vi "Video Processor main.vi"() -> ()   [LabVIEW 2018]
uses:
  Video Processor main Core Status Indicator STYP.ctl
  Video Processor main Status STYP.ctl
  Video Processor main Core Status STYP.ctl
  Video Processor main File Status STYP.ctl
  <userlib>/Jet Engineering/JET_QSM/Code/Private/JET_QSM_InvalidOption STYP.ctl
  <userlib>/Jet Engineering/JET_QSM/Code/Private/JET_QSM - Add State [String API].vi
  80037c5a-716f-4bc2-9a3a-c8c93484ebcc.vi
  35257932-e252-4286-8d59-1e758d2cb38c.vi
  <vilib>/Utility/error.llb/Trim Whitespace.vi
  <vilib>/Utility/error.llb/Error Cluster From Error Code.vi
panel:
  out "Core Statuses":T1[](array[typedef]) {"Progress" scale=0.0..100.0}
  out "Converting?":bool
  out "Progress":dbl(slide) scale=0.0..100.0
  in  "Convert":bool
  in  "Folder":path
  out "Recent states before Error (with tick counts) 2":string="0.167 sec ago: VI Initialize\n0.167 sec ago: Window Open\n0.110 sec ago: Control Update\n0.110 sec ago: Indicator Update\n0.000 sec ago: Error Handler\r\n"
  out "error out":errorcluster
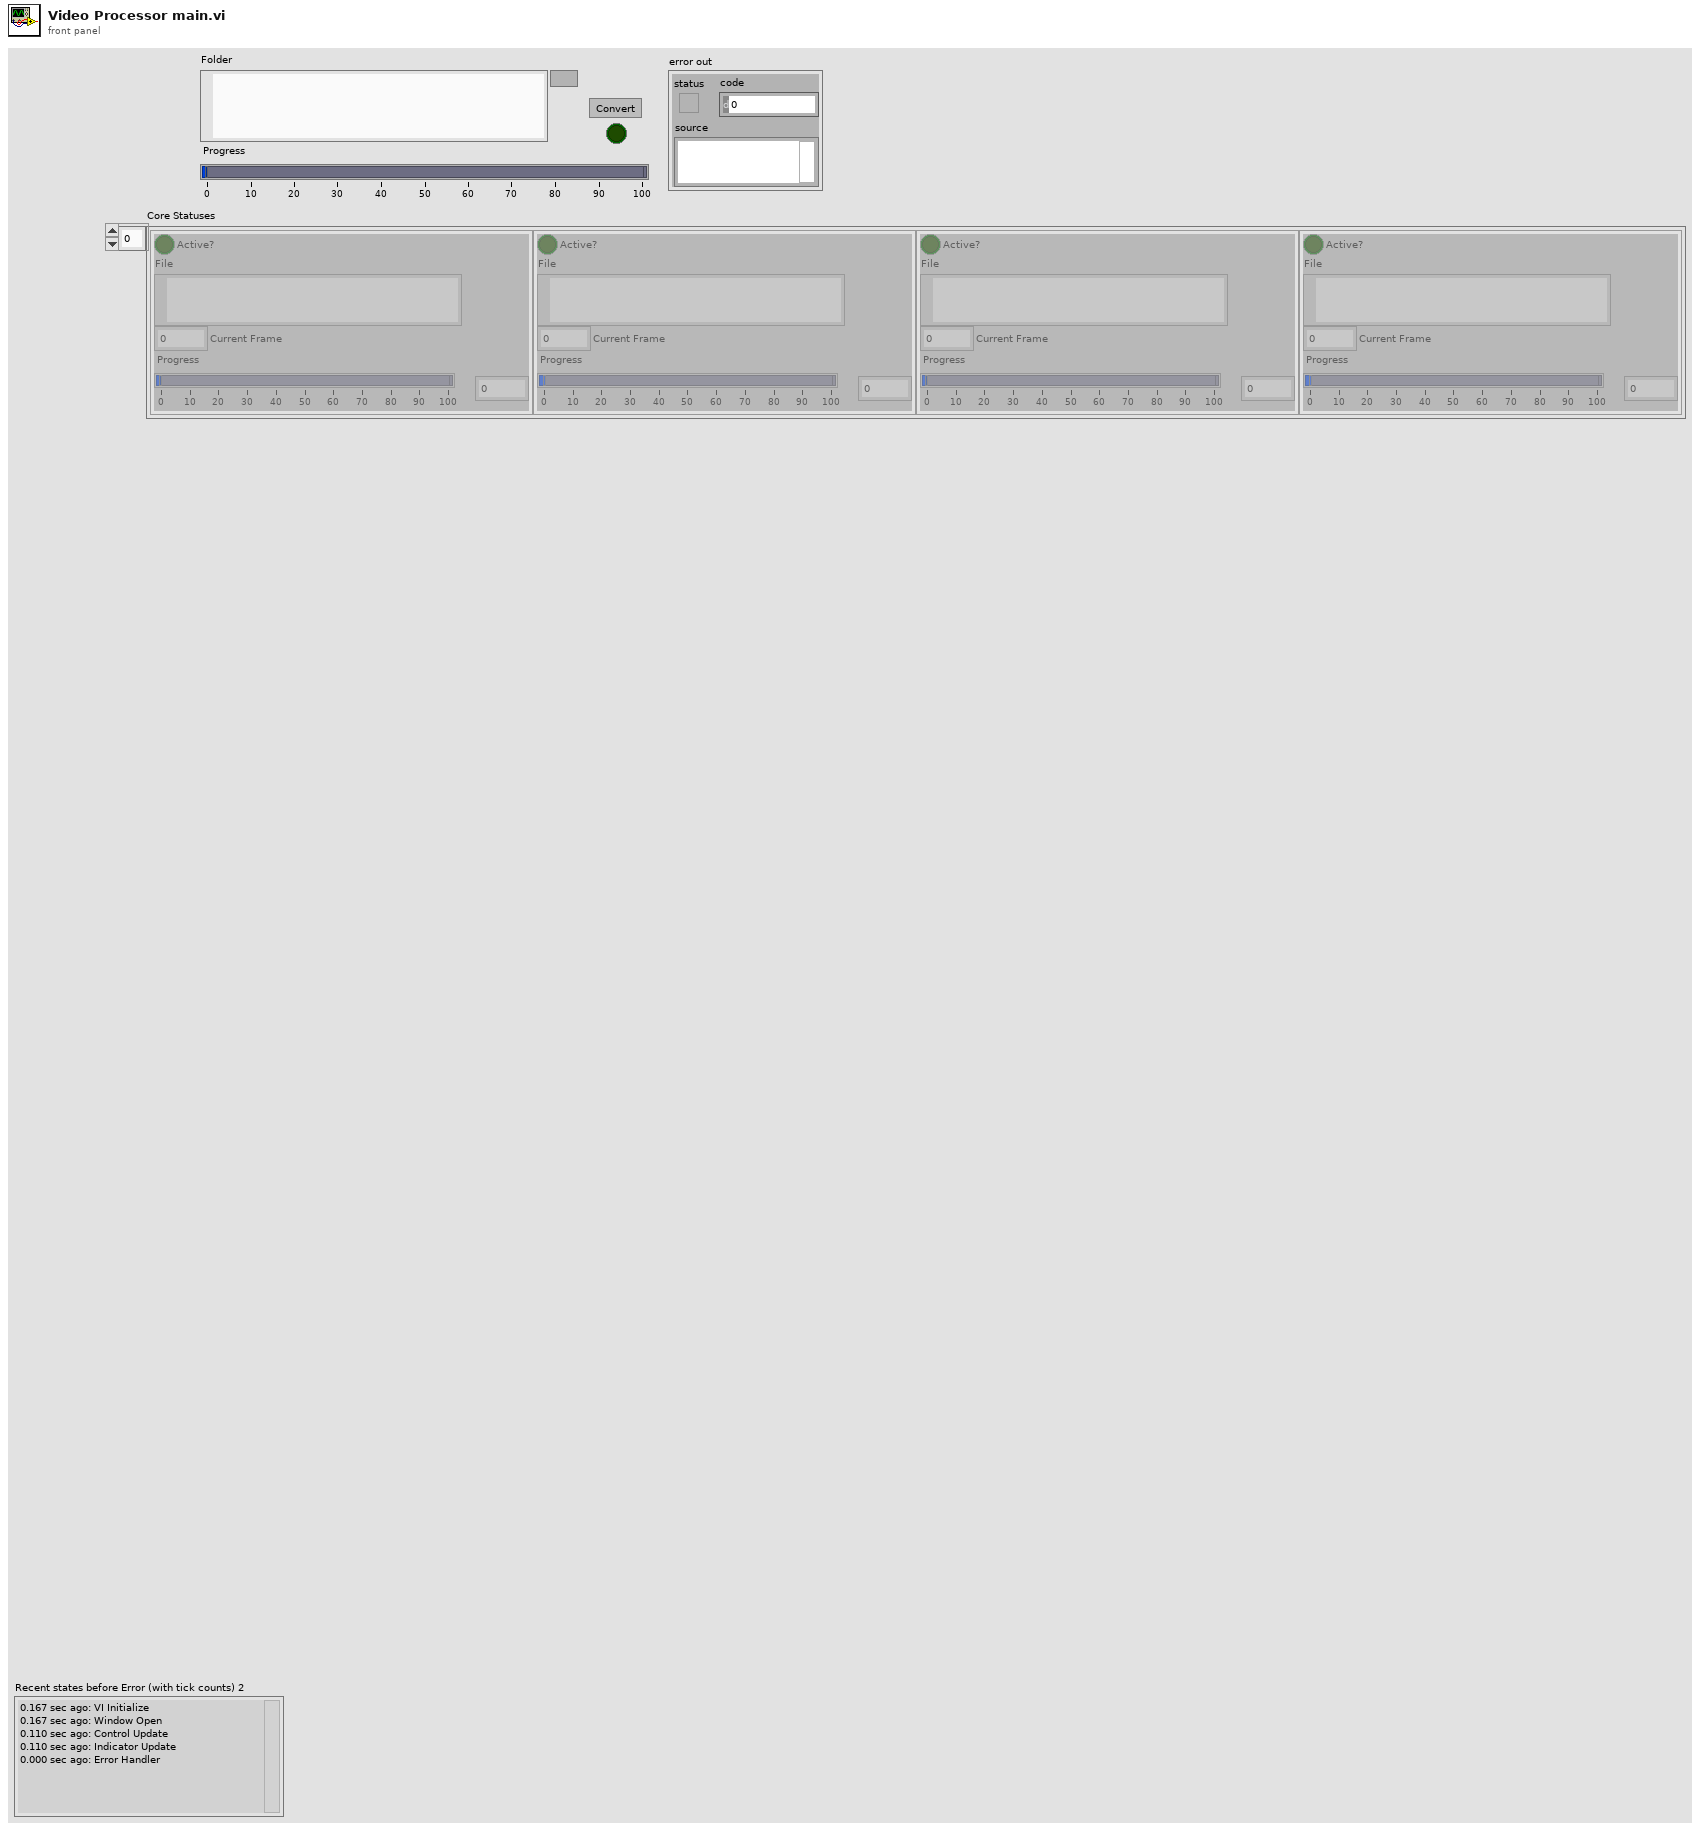
[diagram p1: front panel]
types:
  T1 = typedef "Video Processor main Core Status Indicator STYP.ctl" = cluster{"Active?":bool, "File":path, "Current Frame":i32, "Progress":dbl}
  T2 = typedef "Video Processor main Status STYP.ctl" = cluster{"VI":cluster{"error":errorcluster, "isExiting?":bool}, "UserLoggedIn?":bool, "Converting?":bool, "Input Folder":path, "Files":path[], "Files Complete":i32, "Total File Count":i32, "Core Status":T3[], "Events":cluster{"Refnum":refnum<event-registration>, "Core Release Event":refnum<user-event>, "File Status Event":refnum<user-event>}}
  T3 = typedef "Video Processor main Core Status STYP.ctl" = cluster{"Active?":bool, "File":path, "Current Frame":u32, "Total Frames":u32}
  T4 = typedef "JET_QSM_InvalidOption STYP.ctl" = enum16{"Ignore", "Dialog", "Error"}
  T5 = typedef "JET_QSM_Refnum STYP.ctl" = cluster{"state":cluster{"queue":refnum<queue>, "idle":string, "error":string, "STOP":string}, "debug":cluster{"enabled?":bool, "queue":refnum<queue>}, "Invalid.option":T4, "QSM.Name":string}
  T6 = enum32{"invalid app kind", "Development System", "Run Time System", "Student Edition", "Embedded LabVIEW", "Evaluation", "Custom"}
  T7 = typedef "Video Processor main File Status STYP.ctl" = cluster{"Index":i32, "Current Frame":u32, "Total Frames":u32}
  T8 = typedef "JET_QSM_Element STYP.ctl" = cluster{"state":string, "data":variant, "comment":string}
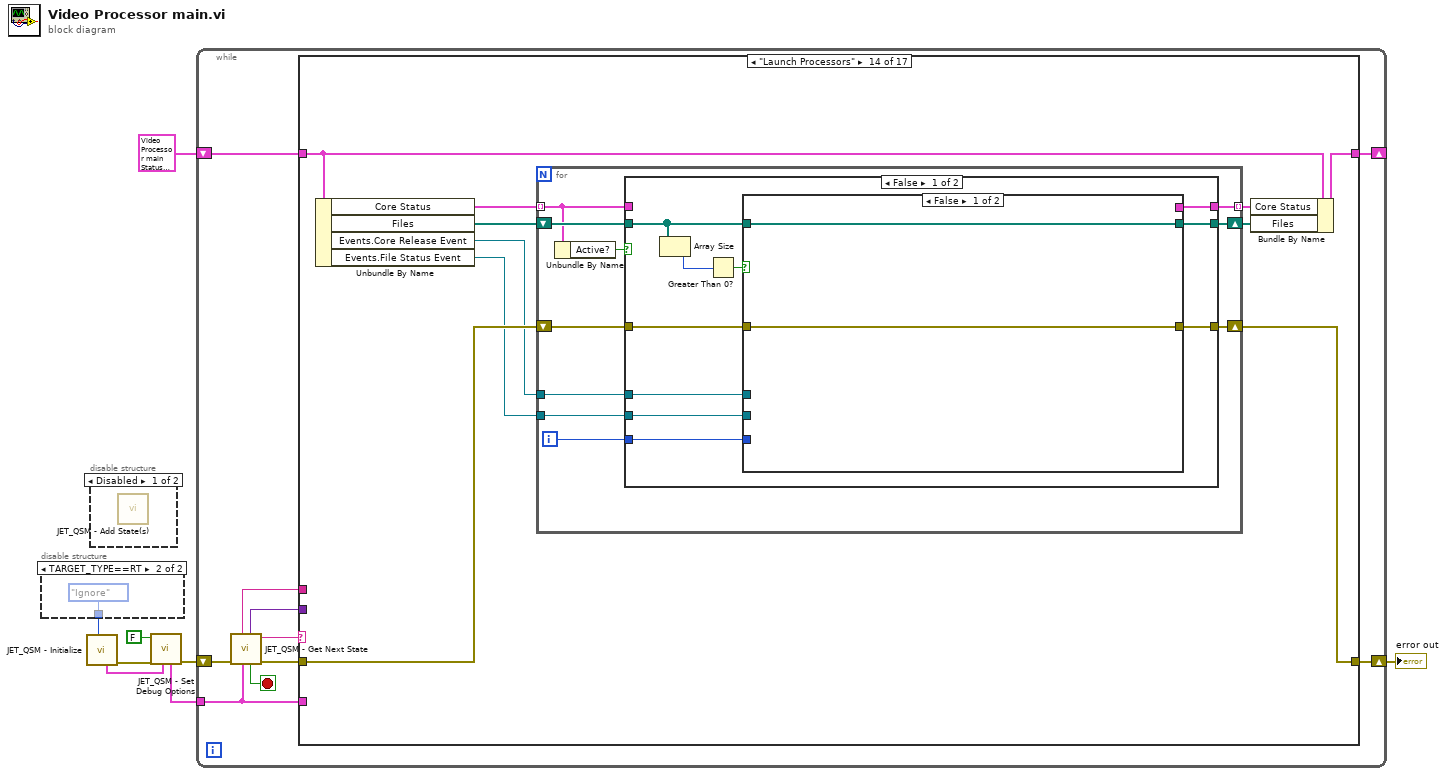
[diagram p0: block diagram]
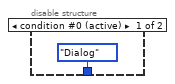
[diagram p2: hidden frame]
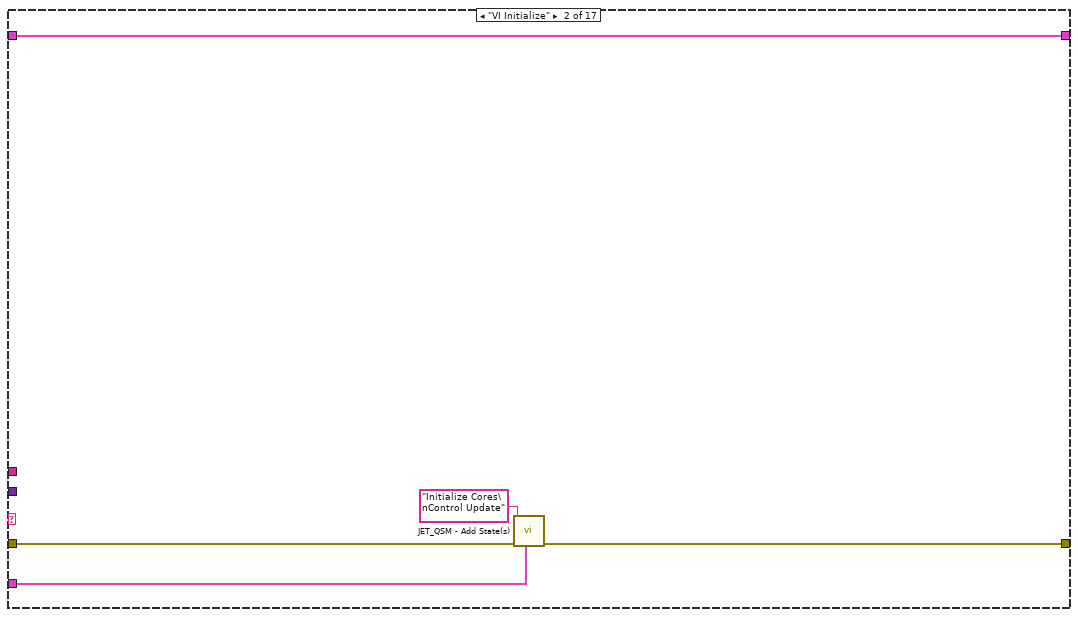
[diagram p5: hidden frame]
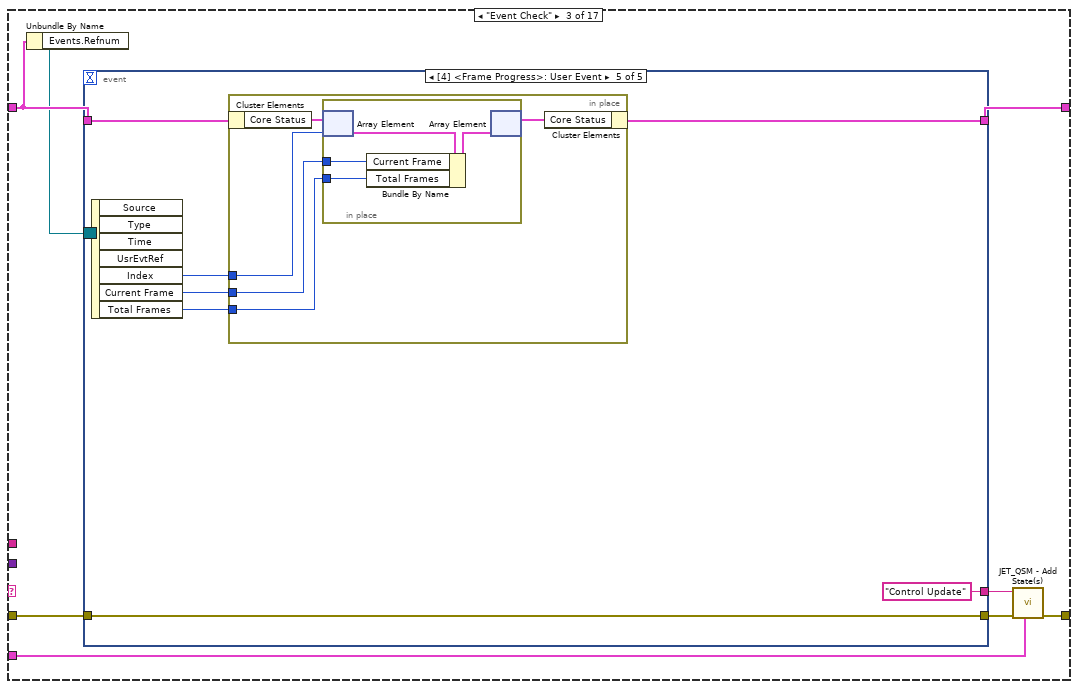
[diagram p6: hidden frame]
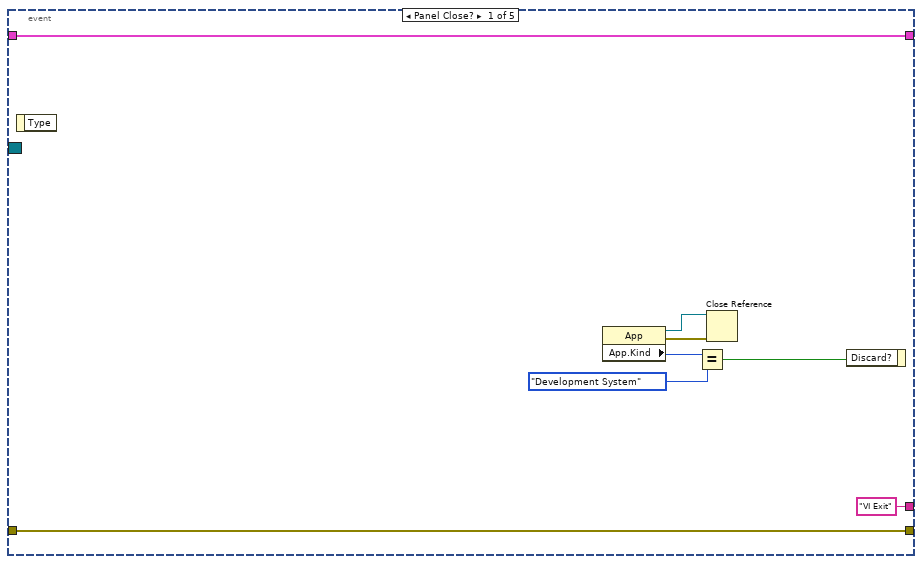
[diagram p7: hidden frame]
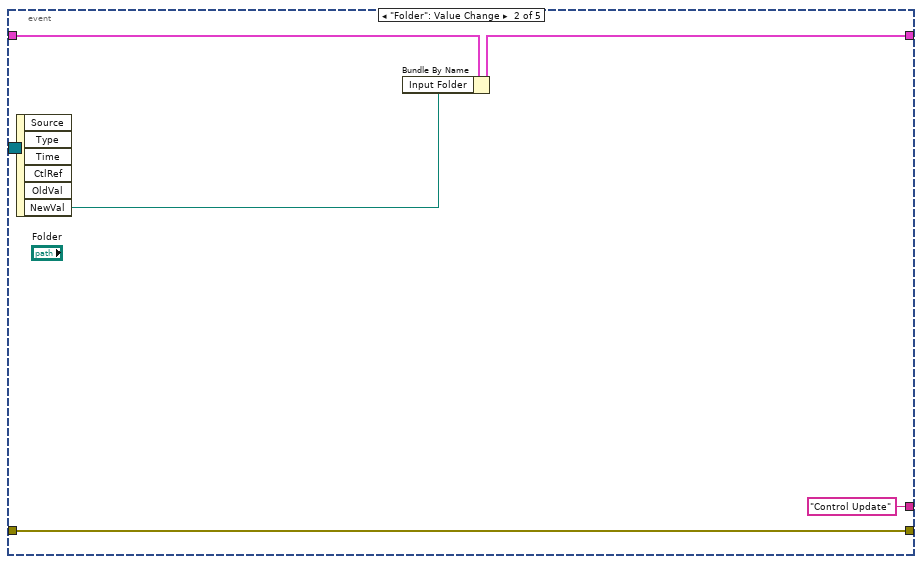
[diagram p8: hidden frame]
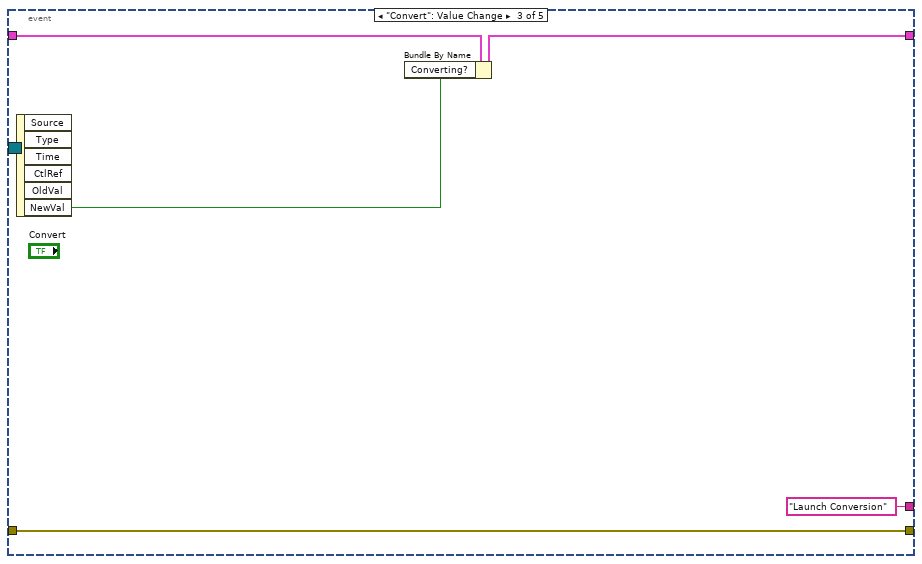
[diagram p9: hidden frame]
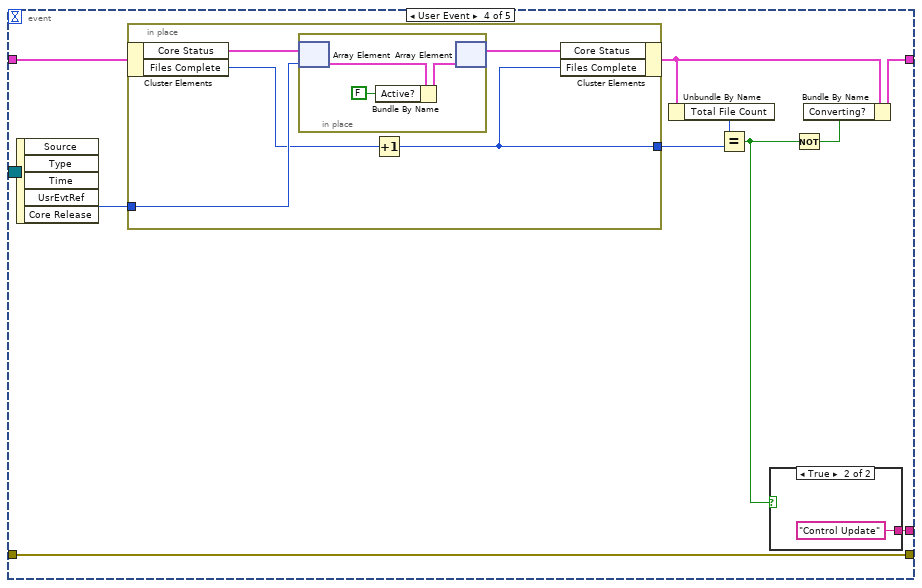
[diagram p10: hidden frame]
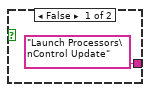
[diagram p11: hidden frame]
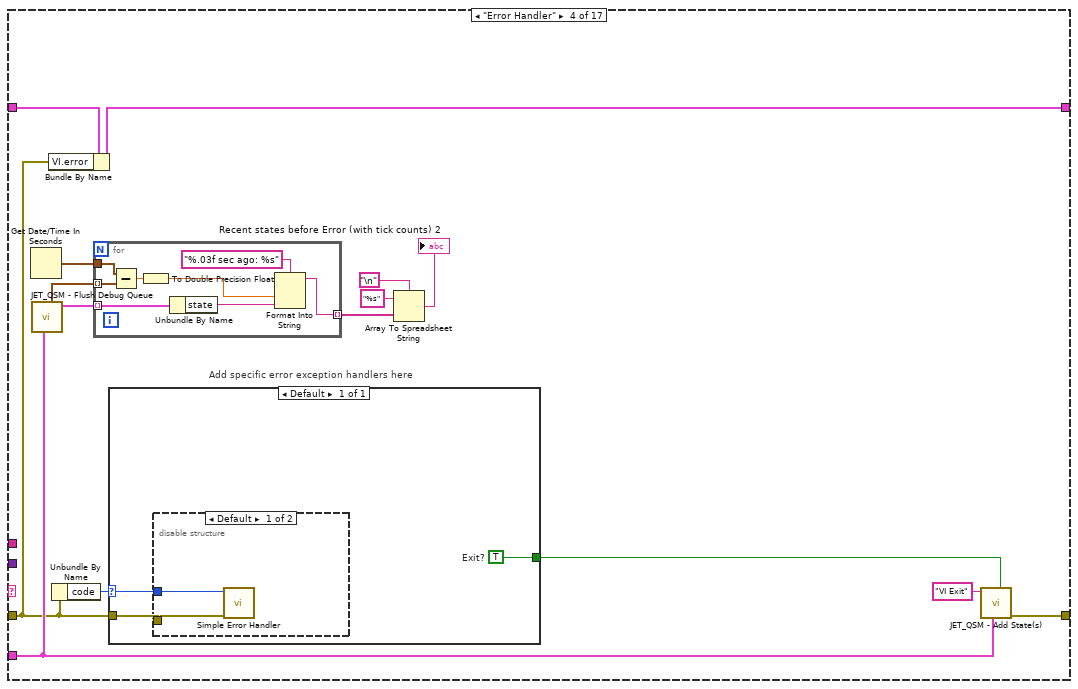
[diagram p12: hidden frame]
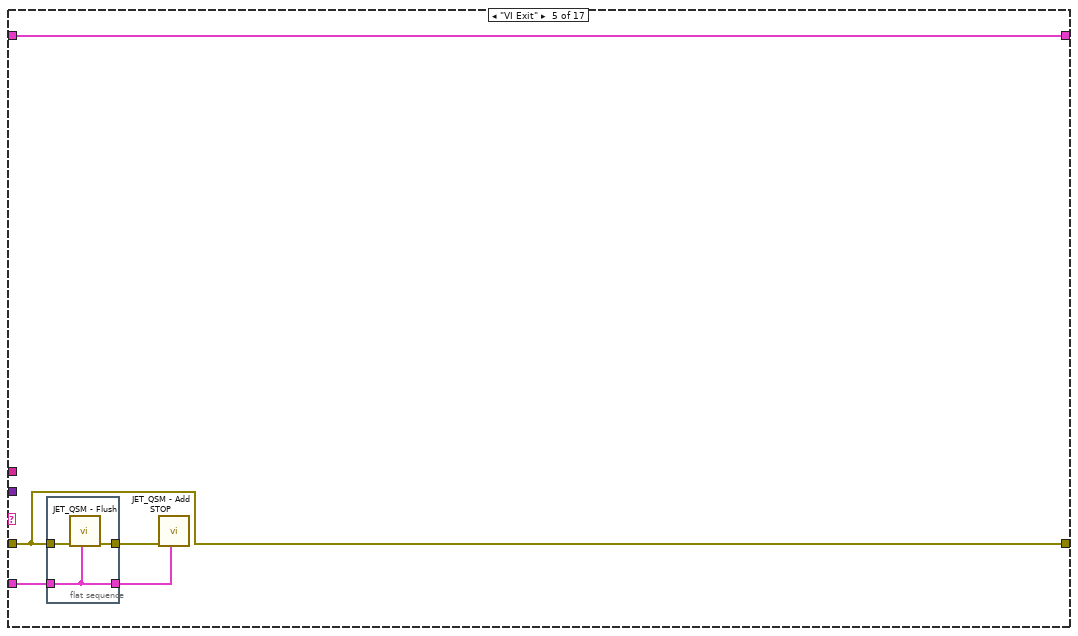
[diagram p14: hidden frame]
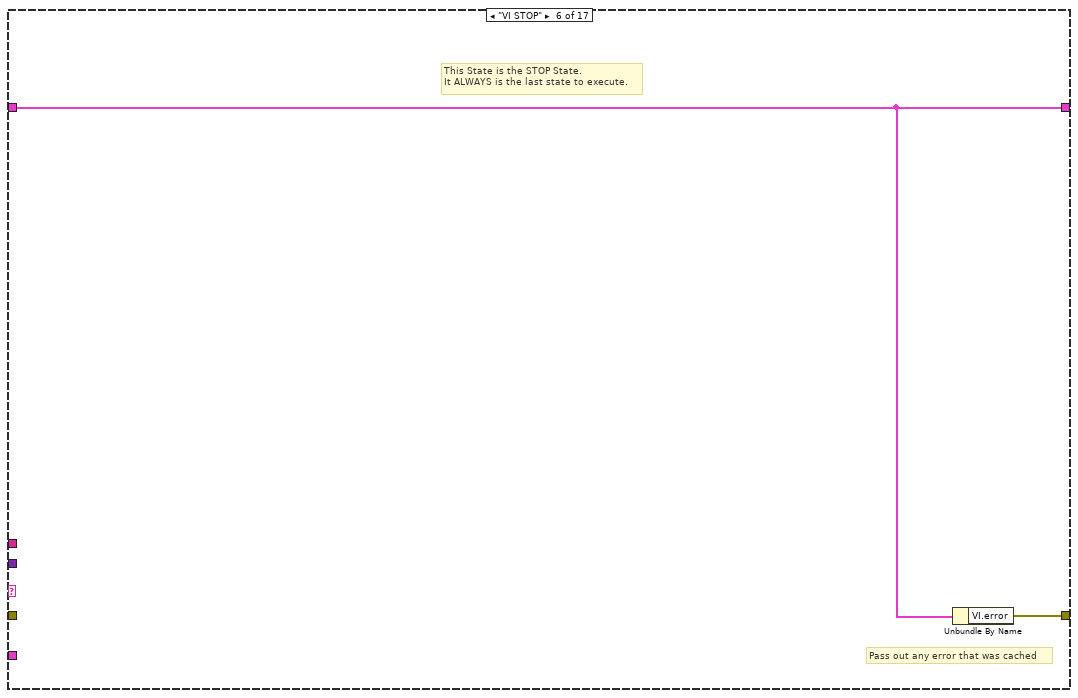
[diagram p15: hidden frame]
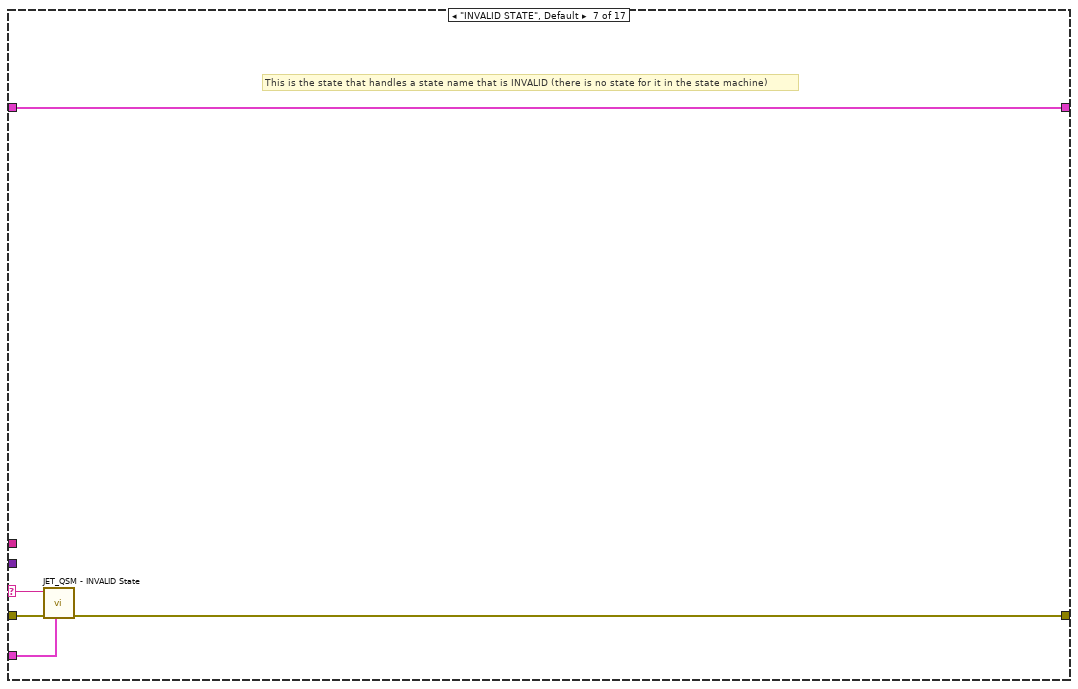
[diagram p16: hidden frame]
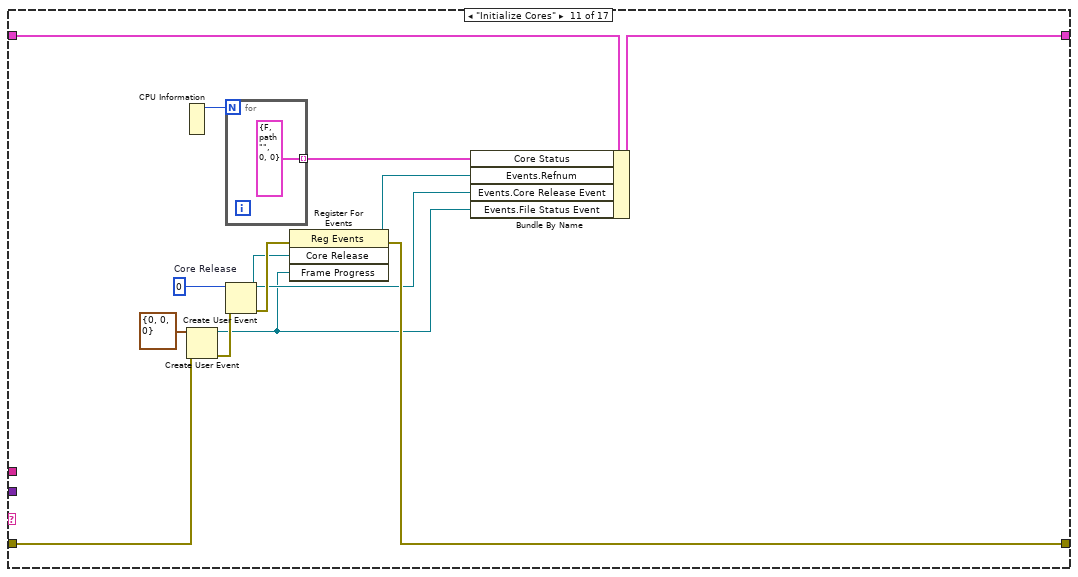
[diagram p20: hidden frame]
diagram:
  n1 = disable-structure shown="TARGET_TYPE==RT" {
    disable-tunnel: [JET_QSM_InvalidOption_STYP."Dialog" ("invalid state action (Dialog)") JET_QSM_InvalidOption_STYP."Ignore" ("invalid state action (Dialog)")] -> w8
    frame condition #0 (active) {
    }
    frame condition #1 {
    }
  }
  n2 = call <userlib>:"JET_QSM - Initialize.vi"("invalid state action (Dialog)"=w8) -> ("error out"=w1:errorcluster, "Jet_QSM refnum"=w4:T5)  [unwired: 9 in]
  n3 = disable-structure shown="Disabled" {
    frame Disabled {
      n4 = call-poly <userlib>:"JET_QSM - Add State(s).vi"() -> ()  [unwired: 11 in, 1 out]
    }
    frame Enabled {
    }
  }
  n5 = call <userlib>:"JET_QSM - Set Debug Options.vi"("Jet_QSM refnum"=w4, "error in (no error)"=w1, "debug.enabled? (F)"=FALSE) -> ("error out"=w2:errorcluster, "Jet_QSM ref"=w3:T5)  [unwired: 7 in]
  n6 = while {
    tunnel: w3 -> [w16]
    shift-right: [w14] -> _
    shift-left: T2 {"VI"={"error"={"status"=FALSE, "code"=0, "source"=""}, "isExiting?"=FALSE}, "UserLoggedIn?"=FALSE, "Converting?"=FALSE, "Input Folder"=path "", "Files"=[], "Files Complete"=0, "Total File Count"=0, "Core Status"=[], "Events"={"Refnum"=refnum, "Core Release Event"=refnum, "File Status Event"=refnum}} ("Status") -> [w15]
    shift-right: [w13] -> w7
    shift-left: w2 -> [w20]
    stop <- w17 stop-if-true
    n7 = call <userlib>:"JET_QSM - Get Next State.vi"("Jet_QSM refnum"=w16, "error in (no error)"=w20) -> ("error out"=w19:errorcluster, "state"=w18:string, "Stop Loop?"=w17:bool, "state data"=w12:variant, "state comment"=w11:string)  [unwired: 5 in]
    n8 = case shown="\"Launch Processors\"" w18 {
      selector: w18 -> [_ _ _ _ _ _ w130 _ _ _ _ _ _ _ _ _ _]
      tunnel: w19 -> [w21 w26 w35 w91 w122 _ w131 w133 w135 w137 w142 w156 w166 w177 w221 w229 w238]
      tunnel: w16 -> [_ w24 w34 w96 w120 _ w129 _ _ _ _ w154 _ _ _ w230 _]
      tunnel: w15 -> [w22 w27 w29 w92 w118 w126 w132 w134 w136 w138 w150 w157 w162 w173 w222 w227 w237]
      tunnel: [w22 w27 w30 w90 w118 w126 w132 w134 w136 w138 w144 w157 w161 w170 w222 w227 w237] -> w14
      tunnel: [w21 w25 w32 w97 w122 w127 w128 w133 w135 w137 w146 w155 w165 w176 w221 w228 w238] -> w13
      tunnel: w12 -> [_ _ _ _ _ _ _ _ _ _ _ _ _ _ _ _ _]
      tunnel: w11 -> [_ _ _ _ _ _ _ _ _ _ _ _ _ _ _ _ _]
      frame "------ Standard States ------" {
        # "Standard States are required states for a JET_QSM State Machine\n\nTheir names may be changed; use the Initialize function to specify the new names"
        # "This is a section header; the state is never expected to execute"
      }
      frame "VI Initialize" {
        n9 = call-poly <userlib>:"JET_QSM - Add State(s).vi"("Jet_QSM refnum"=w24, "error in (no error)"=w26, "state(s)"="Initialize Cores\nControl Update") -> ("error out"=w25:errorcluster)  [unwired: 8 in]
      }
      frame "Event Check" {
        n10 = Unbundle By Name(w29) -> ("Events.Refnum"=w28:refnum<event-registration>)
        n11 = event shown="[4] <Frame Progress>: User Event" {
          selector: w28 -> [_ _ _ _ _]
          dyn-events: _ -> [_ _ _ _ _]
          timeout: _ -> [_ _ _ _ _]
          tunnel: w35 -> [w37 w48 w53 w61 w75]
          tunnel: ["VI Exit" ("state(s)") "Control Update" ("state(s)") "Launch Conversion" ("state(s)") w60 "Control Update" ("state(s)")] -> w33
          tunnel: [w37 w48 w53 w61 w75] -> w31
          tunnel: w29 -> [w36 w46 w51 w63 w80]
          tunnel: [w36 w45 w49 w56 w79] -> w30
          event Panel Close? {
            n12 = event-data() -> ()  [unwired: 1 in, 1 out]
            n13 = property class="App"() -> (reference out=w39:refnum<vi>, error out=w40:errorcluster, "App.Kind"=w43:T6)  [unwired: 2 in]
            n14 = Equal?(x=w43, y=T6."Development System") -> (x = y?=w41:bool)
            n15 = Close Reference(reference=w39, error in (no error)=w40) -> ()  [unwired: 1 out]
            n16 = event-data("Discard?"=w41) -> ()  [unwired: 1 in, 1 out]
          }
          event "Folder": Value Change {
            n17 = event-data() -> ("NewVal"=w44:path)  [unwired: 1 in, 5 out]
            n18 = Bundle By Name(cluster=w46, "Input Folder"=w44) -> (w45:T2)
          }
          event "Convert": Value Change {
            n19 = event-data() -> ("NewVal"=w50:bool)  [unwired: 1 in, 5 out]
            n20 = Bundle By Name(cluster=w51, "Converting?"=w50) -> (w49:T2)
          }
          event User Event {
            n21 = event-data() -> ("Core Release"=w62:i32)  [unwired: 1 in, 4 out]
            n22 = in-place {
              in-place-border: w62 -> [w69]
              in-place-border: [w66] -> w58
              n23 = in-place-cluster #1(w63) -> ("Core Status"=w70:T3[], "Files Complete"=w67:i32)
              n24 = in-place {
                n25 = in-place-array #2(w70, w69) -> (w73:T3)
                n26 = Bundle By Name(cluster=w73, "Active?"=FALSE) -> (w71:T3)
                n27 = in-place-array #2(w71) -> (w68:T3[])  [unwired: 1 out]
              }
              n28 = Increment(x=w67) -> (x+1=w66:i32)
              n29 = in-place-cluster #1("Core Status"=w68, "Files Complete"=w66) -> (w57:T2)
            }
            n30 = Unbundle By Name(w57) -> ("Total File Count"=w59:i32)
            n31 = Equal?(x=w59, y=w58) -> (x = y?=w54:bool)
            n32 = case shown="True" w54 {
              tunnel: ["Launch Processors\nControl Update" ("state(s)") "Control Update" ("state(s)")] -> w60
              frame False {
              }
              frame True {
              }
            }
            n33 = Not(x=w54) -> (.not. x?=w55:bool)
            n34 = Bundle By Name(cluster=w57, "Converting?"=w55) -> (w56:T2)
          }
          event User Event {
            n35 = event-data() -> ("Index"=w78:i32, "Current Frame"=w77:u32, "Total Frames"=w76:u32)  [unwired: 1 in, 4 out]
            n36 = in-place {
              in-place-border: w78 -> [w83]
              in-place-border: w77 -> [w82]
              in-place-border: w76 -> [w81]
              n37 = in-place-cluster #3(w80) -> ("Core Status"=w85:T3[])
              n38 = in-place {
                in-place-border: w82 -> [w88]
                in-place-border: w81 -> [w87]
                n39 = in-place-array #4(w85, w83) -> (w89:T3)
                n40 = Bundle By Name(cluster=w89, "Current Frame"=w88, "Total Frames"=w87) -> (w86:T3)
                n41 = in-place-array #4(w86) -> (w84:T3[])  [unwired: 1 out]
              }
              n42 = in-place-cluster #3("Core Status"=w84) -> (w79:T2)
            }
          }
        }
        n43 = call-poly <userlib>:"JET_QSM - Add State(s).vi"("Jet_QSM refnum"=w34, "error in (no error)"=w31, "state(s)"=w33) -> ("error out"=w32:errorcluster)  [unwired: 8 in]
      }
      frame "Error Handler" {
        # "Add specific error exception handlers here"
        n44 = Get Date/Time In Seconds() -> (seconds since 1Jan1904=w100:timestamp)
        n45 = call <userlib>:"JET_QSM - Flush Debug Queue.vi"("Jet_QSM refnum"=w96) -> ("QSM Elements"=w98:T8[], "Timestamps"=w99:timestamp[])  [unwired: 8 in, 1 out]
        n46 = Bundle By Name(cluster=w92, "VI.error"=w91) -> (w90:T2)
        n47 = Unbundle By Name(w91) -> ("code"=w93:i32)
        n48 = for {
          tunnel: w98 -> [w112] mode=indexing
          tunnel: [w110] -> w102 mode=indexing
          tunnel: w100 -> [w107]
          tunnel: w99 -> [w108] mode=indexing
          n49 = Subtract(x=w107, y=w108) -> (x-y=w106:dbl)
          n50 = To Double Precision Float(number=w106) -> (double precision float=w105:dbl)
          n51 = Unbundle By Name(w112) -> ("state"=w111:string)
          n52 = Format Into String(format string="%.03f sec ago: %s", w105, w111) -> (resulting string=w110:string)  [unwired: 2 in, 1 out]
        }
        n53 = case shown="Default" w93 {
          selector: w93 -> [w114]
          tunnel: [w115] -> w94
          tunnel: w91 -> [w113]
          frame Default {
            w115 = TRUE  # Exit?
            n54 = disable-structure shown="Default" {
              disable-tunnel: w114 -> [w117 _]
              disable-tunnel: w113 -> [w116 _]
              frame condition #0 (active) {
                n55 = call <vilib>:"Simple Error Handler.vi"("error code (no error:0)"=w117, "error in (no error)"=w116) -> ()  [unwired: 3 in, 5 out]
              }
              frame condition #1 {
              }
            }
          }
        }
        n56 = Array To Spreadsheet String(delimiter (Tab)="\n", array=w102, 3:"%s" ("format string")) -> (spreadsheet string=→"Recent states before Error (with tick counts) 2":string)
        n57 = call-poly <userlib>:"JET_QSM - Add State(s).vi"("act? (T)"=w94, "Jet_QSM refnum"=w96, "state(s)"="VI Exit") -> ("error out"=w97:errorcluster)  [unwired: 8 in]
      }
      frame "VI Exit" {
        n58 = flat-sequence {
          tunnel: w122 -> [w125]
          tunnel: [w124] -> w121
          tunnel: w120 -> [w123]
          tunnel: [w123] -> w119
          frame #0 {
            n59 = call <userlib>:"JET_QSM - Flush.vi"("Jet_QSM ref"=w123, "error in (no error)"=w125) -> ("error out"=w124:errorcluster)  [unwired: 8 in, 1 out]
          }
        }
        n60 = call <userlib>:"JET_QSM - Add STOP.vi"("Jet_QSM refnum"=w119, "error in (no error)"=w121) -> ()  [unwired: 9 in, 1 out]
      }
      frame "VI STOP" {
        # "Pass out any error that was cached"
        # "This State is the STOP State.\nIt ALWAYS is the last state to execute."
        n61 = Unbundle By Name(w126) -> ("VI.error"=w127:errorcluster)
      }
      frame "INVALID STATE", Default {
        # "This is the state that handles a state name that is INVALID (there is no state for it in the state machine)"
        n62 = call <userlib>:"JET_QSM - INVALID State.vi"("Jet_QSM refnum"=w129, "error in (no error)"=w131, "state"=w130) -> ("error out"=w128:errorcluster)  [unwired: 8 in]
      }
      frame "------ Menu Commands ------" {
        # "This is a section header; the state is never expected to execute"
      }
      frame "------ Events  ------" {
        # "This is a section header; the state is never expected to execute"
      }
      frame "------ Actions  ------" {
        # "This is a section header; the state is never expected to execute"
      }
      frame "Initialize Cores" {
        w148 = 0  # Core Release
        n63 = CPU Information() -> (4:w151:i32)  [unwired: 3 out]
        n64 = Create User Event(user event datatype=T7 {"Index"=0, "Current Frame"=0, "Total Frames"=0} ("Frame Progress"), error in=w142) -> (user event=w139:refnum<user-event>, error out=w141:errorcluster)
        n65 = for {
          N: w151 -> [_]
          tunnel: [T3 {"Active?"=FALSE, "File"=path "", "Current Frame"=0, "Total Frames"=0} ("Core")] -> w149 mode=indexing
        }
        n66 = Create User Event(user event datatype=w148, error in=w141) -> (user event=w143:refnum<user-event>, error out=w147:errorcluster)
        n67 = register-events(error in=w147, w143, w139) -> (reference out=w145:refnum<event-registration>, error out=w146:errorcluster)  [unwired: 1 in]
        n68 = Bundle By Name(cluster=w150, "Core Status"=w149, "Events.Refnum"=w145, "Events.Core Release Event"=w143, "Events.File Status Event"=w139) -> (w144:T2)
      }
      frame "Launch Conversion" {
        n69 = call-poly <userlib>:"JET_QSM - Add State(s).vi"("Jet_QSM refnum"=w154, "error in (no error)"=w156, "state(s)"="Find Files\nLaunch Processors\nControl Update") -> ("error out"=w155:errorcluster)  [unwired: 8 in]
      }
      frame "Find Files" {
        n70 = Unbundle By Name(w162) -> ("Input Folder"=w164:path)
        n71 = List Folder(path=w164, error in=w166) -> (filenames=w163:string[], error out=w165:errorcluster)  [unwired: 2 in, 2 out]
        n72 = for {
          tunnel: w164 -> [w169]
          tunnel: w163 -> [w168] mode=indexing
          tunnel: [w167] -> w159 mode=indexing
          n73 = Build Path(base path=w169, name or relative path=w168) -> (appended path=w167:path)
        }
        n74 = Array Size(array=w159) -> (size(s)=w160:i32)
        n75 = Bundle By Name(cluster=w162, "Files"=w159, "Files Complete"=1, "Total File Count"=w160) -> (w161:T2)
      }
      frame "Launch Processors" {
        n76 = Unbundle By Name(w173) -> ("Core Status"=w179:T3[], "Files"=w178:path[], "Events.Core Release Event"=w175:refnum<user-event>, "Events.File Status Event"=w174:refnum<user-event>)
        n77 = for {
          tunnel: w179 -> [w187] mode=indexing
          shift-right: [w186] -> w171
          shift-left: w178 -> [w188]
          tunnel: [w185] -> w172 mode=indexing
          shift-right: [w183] -> w176
          shift-left: w177 -> [w184]
          tunnel: w175 -> [w182]
          tunnel: w174 -> [w181]
          i -> [w180]
          n78 = Unbundle By Name(w187) -> ("Active?"=w189:bool)
          n79 = case shown="False" w189 {
            tunnel: w188 -> [w192 w220]
            tunnel: w187 -> [_ w219]
            tunnel: [w199 w220] -> w186
            tunnel: [w193 w219] -> w185
            tunnel: w184 -> [w198 w218]
            tunnel: [w197 w218] -> w183
            tunnel: w182 -> [w195 _]
            tunnel: w181 -> [w196 _]
            tunnel: w180 -> [w194 _]
            frame False {
              n80 = Array Size(array=w192) -> (size(s)=w190:i32)
              n81 = Greater Than 0?(x=w190) -> (x > 0?=w191:bool)
              n82 = case shown="False" w191 {
                tunnel: w192 -> [w201 w217]
                tunnel: [w201 w216] -> w199
                tunnel: w198 -> [w200 w209]
                tunnel: [w200 w208] -> w197
                tunnel: w196 -> [_ w207]
                tunnel: w195 -> [_ w206]
                tunnel: w194 -> [_ w205]
                tunnel: [_ w202] -> w193
                frame False {
                }
                frame True {
                  n83 = Delete From Array(array=w217) -> (deleted portion=w203:path, array with subset deleted=w216:path[])  [unwired: 2 in]
                  n84 = vi-ref "Headless Modular Test W Events.vi"() -> (w212:refnum<vi>)
                  n85 = property class="VI Interface Type 0"(reference=w212, error in=w209) -> (error out=w215:errorcluster, "Path"=w214:path)  [unwired: 1 out]
                  n86 = Open VI Reference(type specifier VI Refnum (for type only)=w212, vi path=w214, options=128, error in (no error)=w215) -> (vi reference=w211:refnum<vi>, error out=w210:errorcluster)  [unwired: 2 in]
                  n87 = call-by-ref "Start Asynchronous Call"(reference=w211, error in=w210, "Core Index"=w205, "File Finished Event"=w206, "File Status Event"=w207, "Path"=w203) -> (error out=w208:errorcluster)  [unwired: 8 in, 1 out]
                  n88 = Bundle By Name(cluster=T3 {"Active?"=TRUE, "File"=path "", "Current Frame"=0, "Total Frames"=100} ("Core"), "File"=w203) -> (w202:T3)
                }
              }
            }
            frame True {
            }
          }
        }
        n89 = Bundle By Name(cluster=w173, "Core Status"=w172, "Files"=w171) -> (w170:T2)
      }
      frame "------ Window and Panel Control ------" {
        # "This is a section header; the state is never expected to execute"
      }
      frame "Control Update" {
        # "Update all control properties here from the status cluster\n(Consolidate/reduce property nodes)"
        n90 = Unbundle By Name(w227) -> ("Input Folder"=w225:path)
        n91 = call <vilib>:"Is Path and Not Empty.vi"("path"=w225) -> ("Is Path and Not Empty?"=w224:bool)  [unwired: 4 in]
        n92 = Not(x=w224) -> (.not. x?=w223:bool)
        n93 = local write "Folder"(w225) -> ()
        n94 = call <userlib>:"VI Control - Disable Control.vi"("Disable? (T)"=w223) -> ("Disabled Attribute"=w226:u8)  [unwired: 7 in, 1 out]
        n95 = property on="Convert" class="Bool"("DisabledEnum"=w226) -> ()  [unwired: 2 in, 2 out]
        n96 = call-poly <userlib>:"JET_QSM - Add State(s).vi"("Jet_QSM refnum"=w230, "error in (no error)"=w229, "state(s)"="Indicator Update") -> ("error out"=w228:errorcluster)  [unwired: 8 in]
      }
      frame "Indicator Update" {
        # "Update all indicator values here from the status cluster\n(Eliminate Local Variables)"
        n97 = Unbundle By Name(w237) -> ("Converting?"=w232:bool, "Files"=w234:path[], "Files Complete"=w236:i32, "Core Status"=w235:T3[])
        "Converting?" <- w232
        n98 = case shown="True" w232 {
          tunnel: w236 -> [_ w248]
          tunnel: w235 -> [_ w247]
          tunnel: w234 -> [_ w242]
          tunnel: [_ w240] -> w233
          frame False {
          }
          frame True {
            n99 = for {
              tunnel: w247 -> [w258] mode=indexing
              tunnel: [w251] -> w246 mode=indexing if=w254
              tunnel: [w249] -> w239 mode=indexing
              n100 = Unbundle By Name(w258) -> ("Active?"=w254:bool, "Current Frame"=w252:u32, "Total Frames"=w257:u32, "File"=w253:path)
              n101 = call "Calculate Percent Complete.vim"("Total"=w257, "Part"=w252) -> ("% Complete"=w250:dbl)
              n102 = Divide(x=w250, y=100.0) -> (x/y=w251:dbl)
              n103 = Bundle By Name(cluster=T1 {"Active?"=FALSE, "File"=path "", "Current Frame"=0, "Progress"=0.0} ("Core Status"), "Active?"=w254, "File"=w253, "Current Frame"=w252, "Progress"=w250) -> (w249:T1)
            }
            "Core Statuses" <- w239
            n104 = Array Size(array=w242) -> (size(s)=w241:i32)
            n105 = To Double Precision Float(number=w248) -> (double precision float=w244:dbl)
            n106 = Add Array Elements(numeric array=w246) -> (sum=w245:dbl)
            n107 = Add(x=w244, y=w245) -> (x+y=w243:dbl)
            n108 = call "Calculate Percent Complete.vim"("Total"=w241, "Part"=w243) -> ("% Complete"=w240:dbl)
          }
        }
        "Progress" <- w233
      }
    }
  }
  "error out" <- w7
